vi "MCLB Initialize.vi"(8 "error in (no error)":errorcluster, 11 "MCLB_Template in":refnum<class "MCLB_Template.lvclass">) -> (0 "error out":errorcluster, 3 "MCLB_Template out":refnum<class "MCLB_Template.lvclass">)   [LabVIEW 2021, in "MCLB_Template.lvclass"]
uses:
  MCLB_Template.lvclass
  MCLB_Template.lvclass/MCLB_Template.ctl
  <userlib>/Control_Lib/MCLB_Lib/MCLB_Lib.lvclass
panel:
  in  "Config_CSV_FilePath":path
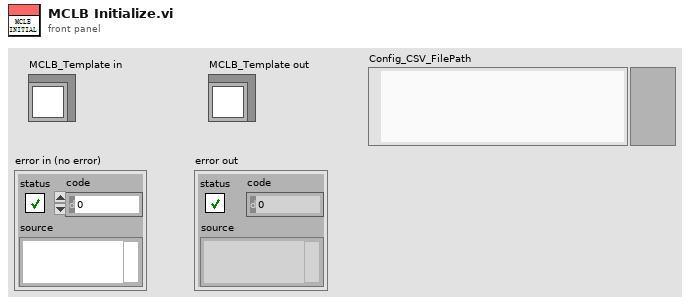
[diagram p1: front panel]
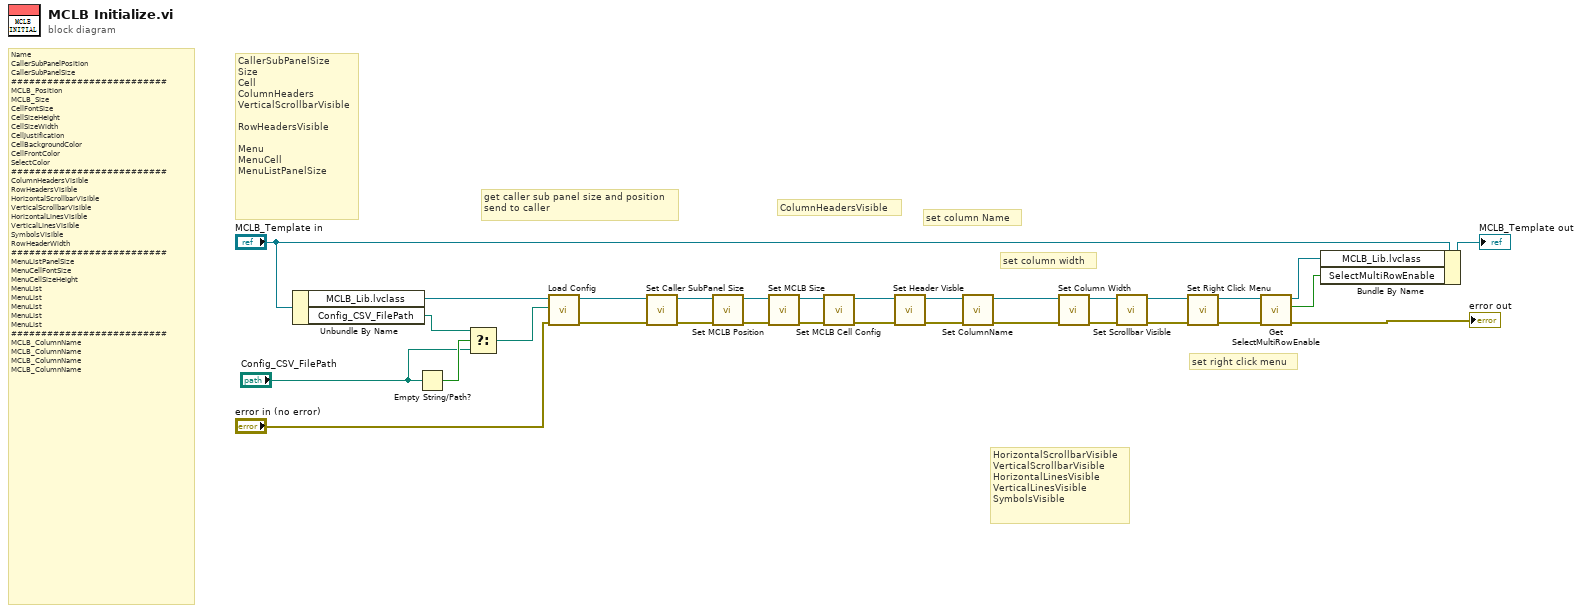
[diagram p0: block diagram]
diagram:
  # "set right click menu"
  # "HorizontalScrollbarVisible\nVerticalScrollbarVisible\nHorizontalLinesVisible\nVerticalLinesVisible\nSymbolsVisible"
  # "set column width"
  # "set column Name"
  # "ColumnHeadersVisible"
  # "get caller sub panel size and position\nsend to caller"
  # "Name\nCallerSubPanelPosition\nCallerSubPanelSize\n##########################\nMCLB_Position\nMCLB_Size\nCellFontSize\nCellSizeHeight\nCellSizeWidth\nCellJustification\nCellBackgroundColor\nCellFrontColor\nSelectColor\n##########################\nColumnHeadersVisible\nRowHeadersVisible\nHorizontalScrollbarVisible\nVerticalScrollbarVisible\nHorizontalLinesVisible\nVerticalLinesVisible\nSymbolsVisible\nRowHeaderWidth\n##########################\nMenuListPanelSize\nMenuCellFontSize\nMenuCellSizeHeight\nMenuList\nMenuList\nMenuList\nMenuList\nMenuList\n##########################\nMCLB_ColumnName\nMCLB_ColumnName\nMCLB_ColumnName\nMCLB_ColumnName"
  # "CallerSubPanelSize\nSize\nCell\nColumnHeaders\nVerticalScrollbarVisible\n\nRowHeadersVisible\n\nMenu\nMenuCell\nMenuListPanelSize"
  n1 = Unbundle By Name("MCLB_Template in") -> ("MCLB_Lib.lvclass"=w7:refnum<class "MCLB_Lib.lvclass">, "Config_CSV_FilePath"=w27:path)
  n2 = Empty String/Path?(string/path="Config_CSV_FilePath") -> (empty?=w29:bool)
  n3 = Select(t=w27, s=w29, f="Config_CSV_FilePath") -> (s? t:f=w26:path)
  n4 = call <userlib>:"Load Config.vi"("error in (no error)"="error in (no error)", "Config_CSV_FilePath"=w26, "MCLB_Lib in"=w7) -> ("error out"=w30:errorcluster, "MCLB_Lib out"=w31:refnum<class "MCLB_Lib.lvclass">)  [unwired: 7 in]
  n5 = call <userlib>:"Set Caller SubPanel Size.vi"("error in (no error)"=w30, "MCLB_Lib in"=w31) -> ("error out"=w24:errorcluster, "MCLB_Lib out"=w25:refnum<class "MCLB_Lib.lvclass">)  [unwired: 6 in, 2 out]
  n6 = call <userlib>:"Set MCLB Position.vi"("error in (no error)"=w24, "MCLB_Lib in"=w25) -> ("error out"=w23:errorcluster, "MCLB_Lib out"=w22:refnum<class "MCLB_Lib.lvclass">)  [unwired: 8 in]
  n7 = call <userlib>:"Set MCLB Size.vi"("error in (no error)"=w23, "MCLB_Lib in"=w22) -> ("error out"=w20:errorcluster, "MCLB_Lib out"=w21:refnum<class "MCLB_Lib.lvclass">)  [unwired: 8 in]
  n8 = call <userlib>:"Set MCLB Cell Config.vi"("error in (no error)"=w20, "MCLB_Lib in"=w21) -> ("error out"=w18:errorcluster, "MCLB_Lib out"=w19:refnum<class "MCLB_Lib.lvclass">)  [unwired: 8 in]
  n9 = call <userlib>:"Set Header Visble.vi"("error in (no error)"=w18, "MCLB_Lib in"=w19) -> ("error out"=w14:errorcluster, "MCLB_Lib out"=w17:refnum<class "MCLB_Lib.lvclass">)  [unwired: 8 in]
  n10 = call <userlib>:"Set ColumnName.vi"("error in (no error)"=w14, "MCLB_Lib in"=w17) -> ("error out"=w15:errorcluster, "MCLB_Lib out"=w16:refnum<class "MCLB_Lib.lvclass">)  [unwired: 8 in]
  n11 = call <userlib>:"Set Column Width.vi"("error in (no error)"=w15, "MCLB_Lib in"=w16) -> ("error out"=w13:errorcluster, "MCLB_Lib out"=w12:refnum<class "MCLB_Lib.lvclass">)  [unwired: 8 in]
  n12 = call <userlib>:"Set Scrollbar Visible.vi"("error in (no error)"=w13, "MCLB_Lib in"=w12) -> ("error out"=w10:errorcluster, "MCLB_Lib out"=w11:refnum<class "MCLB_Lib.lvclass">)  [unwired: 8 in]
  n13 = call <userlib>:"Set Right Click Menu.vi"("error in (no error)"=w10, "MCLB_Lib in"=w11) -> ("error out"=w3:errorcluster, "MCLB_Lib out"=w5:refnum<class "MCLB_Lib.lvclass">)  [unwired: 8 in]
  n14 = call <userlib>:"Get SelectMultiRowEnable.vi"("error in (no error)"=w3, "MCLB_Lib in"=w5) -> ("error out"=→"error out":errorcluster, "SelectMultiRowEnable"=w1:bool, "MCLB_Lib out"=w4:refnum<class "MCLB_Lib.lvclass">)  [unwired: 7 in]
  n15 = Bundle By Name(cluster="MCLB_Template in", "MCLB_Lib.lvclass"=w4, "SelectMultiRowEnable"=w1) -> (→"MCLB_Template out":refnum<class "MCLB_Template.lvclass">)
